vi "File Header.vi"(8 "Settings":string, 9 "Sensors":string, 10 "Locations":string, 11 "Stripped Path":path) -> (3 "File Header":string)   [LabVIEW 2021]
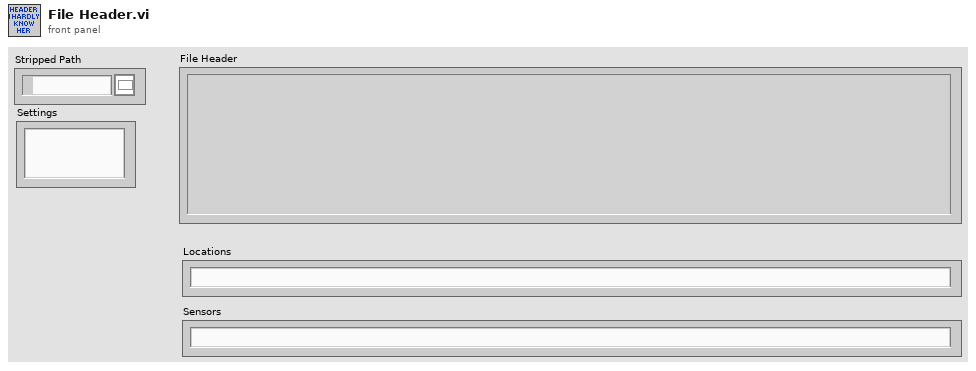
[diagram p1: front panel]
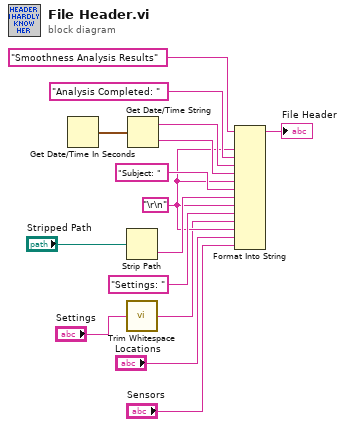
[diagram p0: block diagram]
diagram:
  w5 = "\r\n"
  n1 = Get Date/Time In Seconds() -> (seconds since 1Jan1904=w10:timestamp)
  n2 = Strip Path(path="Stripped Path") -> (name=w7:string)  [unwired: 1 out]
  n3 = call <vilib>:"Trim Whitespace.vi"("string"="Settings") -> ("trimmed string"=w3:string)  [unwired: 1 in]
  n4 = Get Date/Time String(seconds (now)=w10) -> (date string=w13:string, time string=w14:string)  [unwired: 2 in]
  n5 = Format Into String(initial string="Smoothness Analysis Results", w5, "Analysis Completed: " ("input 2"), w13, w14, w5, "Subject: " ("input 6"), w7, w5, "Settings: " ("input 9"), w3, w5, "Locations", "Sensors") -> (resulting string=→"File Header":string)  [unwired: 2 in, 1 out]
